vi "Create Logger.vi"(7 "Level":T1, 8 "error in (no error)":errorcluster, 10 "Options":T2={"filesize (bytes)"=5000000, "logs max age (days) "=10, "write per N messages"=1}, 11 "Root Logging Path":path) -> (0 "error out":errorcluster)   [LabVIEW 2016, in "Global_logger.lvlib"]
uses:
  Global_logger.lvlib
  Options.ctl
  Levels.ctl
  Event.ctl
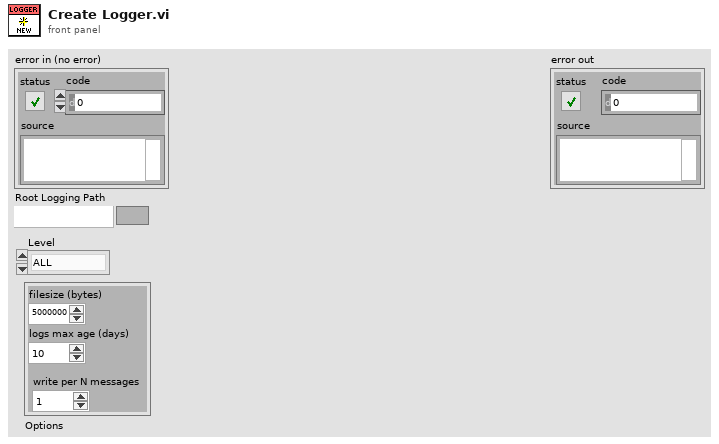
[diagram p1: front panel]
types:
  T1 = typedef "Global_logger.lvlib/Levels.ctl" = enum16{"ALL", "TRACE", "DEBUG", "INFO", "WARN", "ERROR", "FATAL", "OFF"}
  T2 = typedef "Global_logger.lvlib/Options.ctl" = cluster{"filesize (bytes)":u32, "logs max age (days) ":u16, "write per N messages":u16}
  T3 = typedef "Global_logger.lvlib/Event.ctl" = cluster{"Time Stamp":timestamp, "Level":T1, "Source":string, "Message":string}
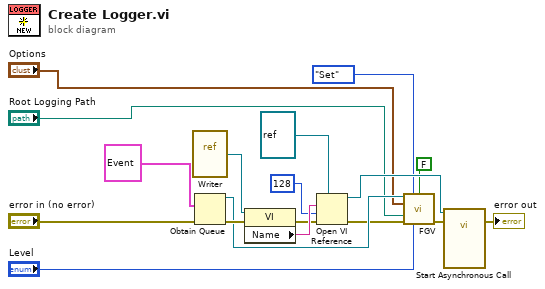
[diagram p0: block diagram]
diagram:
  n1 = vi-ref "Writer.vi"() -> (w18:refnum<vi>)
  n2 = Obtain Queue(element data type=T3 {"Time Stamp"=timestamp(0 s since 1904-01-01), "Level"=enum."ALL", "Source"="", "Message"=""} ("Event"), error in (no error)="error in (no error)") -> (queue out=w8:refnum<queue>, error out=w10:errorcluster)  [unwired: 3 in, 1 out]
  n3 = property class="VI"(reference=w18, error in=w10) -> (error out=w14:errorcluster, "Name"=w17:string)  [unwired: 1 out]
  n4 = Open VI Reference(type specifier VI Refnum (for type only)=refnum<vi> refnum, vi path=w17, options=128, error in (no error)=w14) -> (vi reference=w15:refnum<vi>, error out=w4:errorcluster)  [unwired: 2 in]
  n5 = call "FGV.vi"("queue in"=w8, "Action"=enum16{"Get", "Set"}."Set", "Destroy Logger in"=FALSE, "Options in"="Options", "Root Logging Path in"="Root Logging Path", "error in (no error)"=w4, "Level in"="Level") -> ("error out"=w3:errorcluster)  [unwired: 3 in, 5 out]
  n6 = call-by-ref "Start Asynchronous Call"(reference=w15, error in=w3) -> (error out=→"error out":errorcluster)  [unwired: 12 in, 1 out]
